vi "Init.vi"() -> (3 "Setup Msg Strategy out":refnum<class "Setup Msg Strategy.lvclass">)   [LabVIEW 2021, in "Setup Msg Strategy.lvlib" / "Setup Msg Strategy.lvclass"]
uses:
  Setup Msg Strategy.lvclass
  Setup Msg Strategy.lvclass/Setup Msg Strategy.ctl
  jettl/Sender/Sender.lvlib
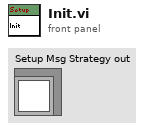
[diagram p1: front panel]
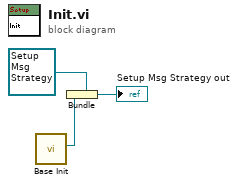
[diagram p0: block diagram]
diagram:
  n1 = call "Base Init.vi"() -> ("Sender"=w1:refnum<class "Sender.lvclass">)  [unwired: 11 in]
  n2 = Bundle "Bundle"(cluster=refnum<class "Setup Msg Strategy.lvclass"> refnum ("Setup Msg out"), w1) -> (→"Setup Msg Strategy out":refnum<class "Setup Msg Strategy.lvclass">)
